vi "GroundRemoval.vi"(0 "Noise high cutoff, Hz":dbl=10000.0 format="%#_13g", 1 "Sampling rate, Hz":dbl=100000.0 format="%#_13g", 5 "Noise filter ratio":dbl=0.9 format="%#_13g", 7 "Number of samplings":i32=10000, 9 "Ground level BP-filter width, Hz":dbl format="%#_13g", 11 "Generator frequency, Hz":dbl format="%#_13g", 12 "Slide":dbl(slide) scale=-2.5..2.5) -> (4 "Final array size":i32, 6 "Final Waveform":dbl[](array[numeric]), 8 "Field":dbl[](array[numeric]), 10 "Time":dbl[](array[numeric]))   [LabVIEW 2015]
uses:
  <vilib>/Analysis/baseanly.llb/Mean (DBL).vi
  <vilib>/Analysis/NI_AALBase.lvlib
panel:
  out "Noise low cutoff, Hz":dbl format="%#_13g"
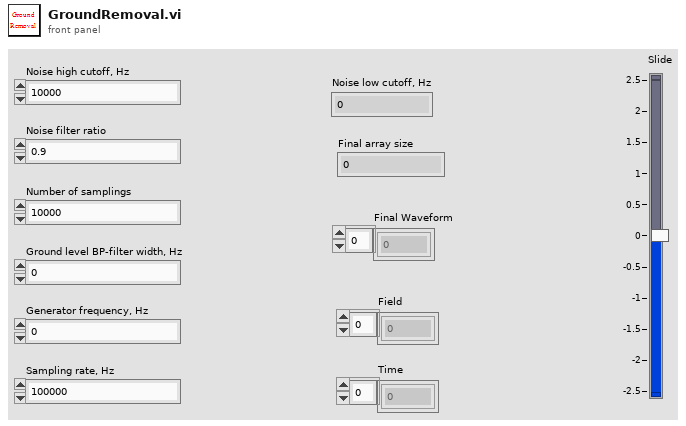
[diagram p1: front panel]
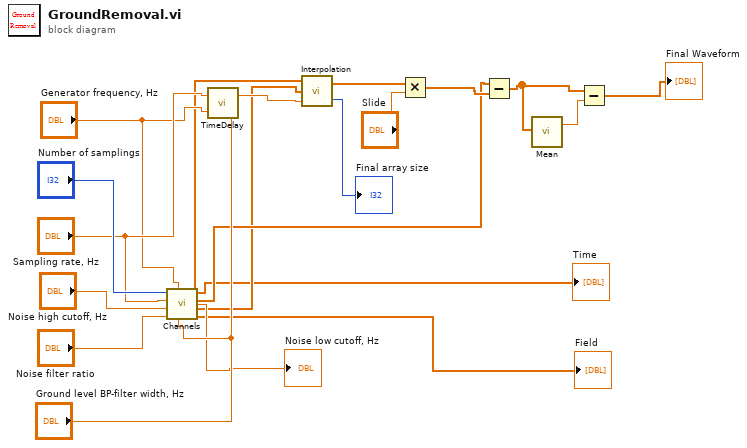
[diagram p0: block diagram]
diagram:
  n1 = call "Channels.vi"("Ground level BP-filter width, Hz"="Ground level BP-filter width, Hz", "Generator frequency, Hz"="Generator frequency, Hz", "Noise filter ratio"="Noise filter ratio", "Noise high cutoff, Hz"="Noise high cutoff, Hz", "Sampling rate, Hz"="Sampling rate, Hz", "Number of samplings"="Number of samplings") -> ("Field"=→"Field":dbl[], "Background"=w8:dbl[], "Differential"=w9:dbl[], "Time"=w5:dbl[], "Noise low cutoff"=→"Noise low cutoff, Hz":dbl)
  "Time" <- w5
  n2 = call "TimeDelay.vi"("Ground level BP-filter width, Hz"="Ground level BP-filter width, Hz", "Generator frequency"="Generator frequency, Hz", "Sampling frequency"="Sampling rate, Hz") -> ("dt"=w10:dbl)
  n3 = call "Interpolation.vi"("dt"=w10, "Shifted Y"=w8, "Original X"=w5) -> ("k"=→"Final array size":i32, "Recovered Y"=w18:dbl[])
  n4 = Multiply(x=w18, y="Slide") -> (x*y=w17:dbl[])
  n5 = Subtract(x=w9, y=w17) -> (x-y=w3:dbl[])
  n6 = call-poly <vilib>:"Mean.vi"("X"=w3) -> ("mean"=w2:dbl)  [unwired: 1 out]
  n7 = Subtract(x=w3, y=w2) -> (x-y=→"Final Waveform":dbl[])
